vi "COM_Port_FGV.vi"(2 "error in (no error)":errorcluster, 3 "COM Port In":refnum<visa-resource-name>="NI_USB_485", 4 "Action":T1=enum."R") -> (0 "error out":errorcluster, 1 "COM Port Out":refnum<visa-resource-name>="NI_USB_485")   [LabVIEW 2018]
uses:
  CTL/FGV - R-W.ctl
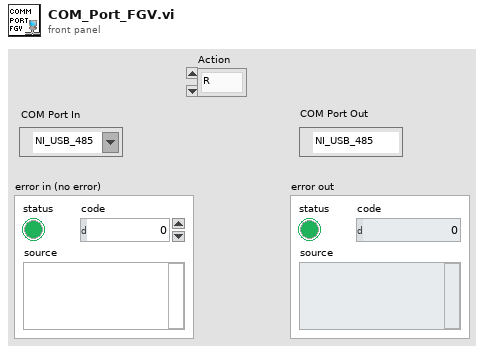
[diagram p1: front panel]
types:
  T1 = typedef "FGV - R-W.ctl" = enum16{"W", "R"}
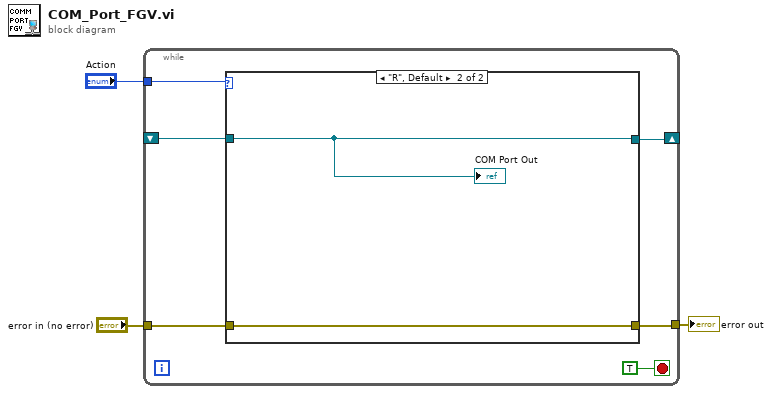
[diagram p0: block diagram]
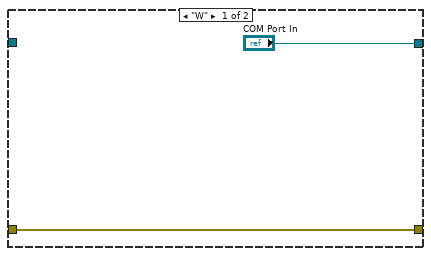
[diagram p2: hidden frame]
diagram:
  n1 = while {
    tunnel: "Action" -> [w8]
    tunnel: [w7] -> w1
    tunnel: "error in (no error)" -> [w6]
    shift-right: [w5] -> _
    shift-left: _ -> [w4]
    stop <- TRUE stop-if-true
    n2 = case shown="\"R\", Default" w8 {
      tunnel: [w11 w13] -> w7
      tunnel: w6 -> [w11 w13]
      tunnel: ["COM Port In" w12] -> w5
      tunnel: w4 -> [_ w12]
      frame "W" {
      }
      frame "R", Default {
        "COM Port Out" <- w12
      }
    }
  }
  "error out" <- w1
